vi "Release Msg Q.vi"(11 "Msg Queue in":refnum<class "Msg Q.lvclass">) -> (0 "error out":errorcluster, 2 "Remaining Elements":refnum<class "Msg.lvclass">[](array[class]))   [LabVIEW 2021, in "AAM.lvlib" / "Msg Q.lvclass"]
uses:
  Msg Q.lvclass
  Msg/Msg.lvclass
  Msg Q.lvclass/Msg Q.ctl
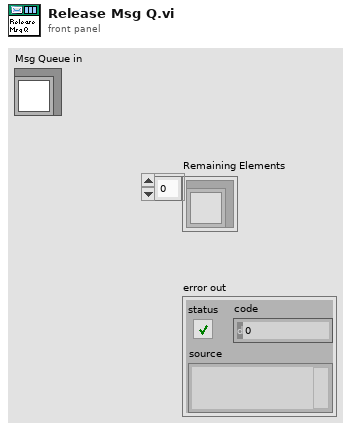
[diagram p1: front panel]
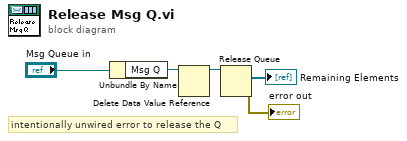
[diagram p0: block diagram]
diagram:
  # "intentionally unwired error to release the Q"
  n1 = Unbundle By Name("Msg Queue in") -> ("Msg Q"=w4:refnum<data-value>)
  n2 = Delete Data Value Reference(data value reference=w4) -> (data value=w3:refnum<queue>)  [unwired: 1 in, 1 out]
  n3 = Release Queue(queue=w3) -> (remaining elements=→"Remaining Elements":refnum<class "Msg.lvclass">[], error out=→"error out":errorcluster)  [unwired: 2 in, 1 out]
